vi "Get Edge Cost.vi"(8 "error in (no error)":errorcluster, 9 "end node":string, 10 "start node":string, 11 "map reference in":refnum<data-value>) -> (0 "error out":errorcluster, 1 "found?":bool, 2 "cost":dbl, 3 "map reference out":refnum<data-value>)   [LabVIEW 2017, in "NI_Robotics_DirectedGraphWorldMap.lvclass"]
doc: "Returns the cost of traversing the edge, or area, of the directed graph map between <B>start node</B> and <B>end node</B>."
uses:
  <vilib>/robotics/Navigation/shared/WorldMap/DirectedGraphWorldMap/NI_Robotics_DirectedGraphWorldMap.lvclass
  <vilib>/robotics/Navigation/shared/MapNode/DirectedGraphMapNode/NI_Robotics_DirectedGraphMapNode.lvclass
  c:/Program Files (x86)/National Instruments/LabVIEW 2017/vi.lib/robotics/Navigation/shared/MapNode/AbstractMapNode/NI_Robotics_AbstractMapNode.lvclass
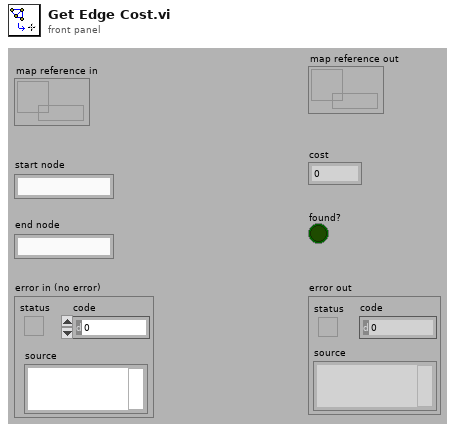
[diagram p1: front panel]
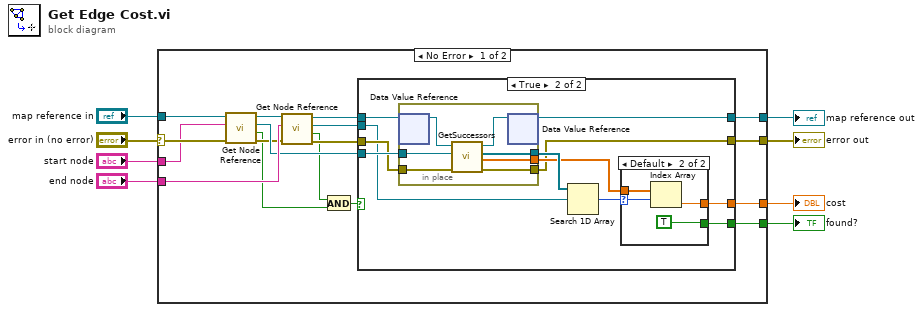
[diagram p0: block diagram]
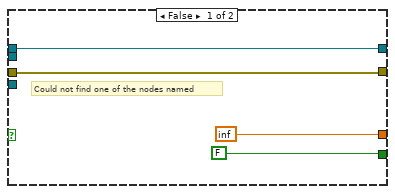
[diagram p2: hidden frame]
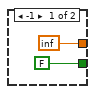
[diagram p3: hidden frame]
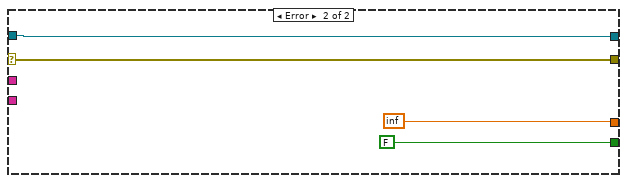
[diagram p4: hidden frame]
diagram:
  n1 = case shown="No Error" "error in (no error)" {
    selector: "error in (no error)" -> [w24 w56]
    tunnel: "map reference in" -> [w25 w57]
    tunnel: "start node" -> [w23 _]
    tunnel: "end node" -> [w21 _]
    tunnel: [w12 w57] -> w2
    tunnel: [w11 inf] -> w4
    tunnel: [w10 w56] -> w5
    tunnel: [w9 FALSE ("found?")] -> w1
    frame No Error {
      n2 = call <vilib>:"Get Node Reference.vi"("error in (no error)"=w24, "name"=w23, "map reference in"=w25) -> ("error out"=w17:errorcluster, "found?"=w13:bool, "node reference"=w19:refnum<data-value>, "map reference out"=w22:refnum<data-value>)  [unwired: 5 in]
      n3 = call <vilib>:"Get Node Reference.vi"("error in (no error)"=w17, "name"=w21, "map reference in"=w22) -> ("error out"=w16:errorcluster, "found?"=w14:bool, "node reference"=w18:refnum<data-value>, "map reference out"=w20:refnum<data-value>)  [unwired: 5 in]
      n4 = And(x=w14, y=w13) -> (x .and. y?=w15:bool)
      n5 = case shown="True" w15 {
        tunnel: w20 -> [w29 w33]
        tunnel: w19 -> [_ w40]
        tunnel: w18 -> [_ w34]
        tunnel: w16 -> [w26 w39]
        tunnel: [w26 w30] -> w10
        tunnel: [w29 w32] -> w12
        tunnel: [inf w35] -> w11
        tunnel: [FALSE ("found?") w31] -> w9
        frame False {
          # "Could not find one of the nodes named"
        }
        frame True {
          n6 = in-place {
            in-place-border: w40 -> [w47]
            in-place-border: w39 -> [w46]
            in-place-border: [w45] -> w30
            in-place-border: [w44] -> w37
            in-place-border: [w43] -> w36
            n7 = in-place-dvr #1(w33) -> (w42:refnum<class "NI_Robotics_DirectedGraphWorldMap.lvclass">)  [unwired: 1 out]
            n8 = call-dynamic "GetSuccessors.vi"("error in (no error)"=w46, "AbstractMapNode Ref"=w47, "WorldMap in"=w42) -> ("error out"=w45:errorcluster, "EdgeCost"=w43:dbl[], "Successors"=w44:refnum<data-value>[], "WorldMap out"=w41:refnum<class "NI_Robotics_DirectedGraphWorldMap.lvclass">)  [unwired: 5 in]
            n9 = in-place-dvr #1(w41) -> (w32:refnum<data-value>)  [unwired: 1 out]
          }
          n10 = Search 1D Array(1D array=w37, element=w34) -> (index of element=w38:i32)  [unwired: 1 in]
          n11 = case shown="Default" w38 {
            selector: w38 -> [_ w53]
            tunnel: w36 -> [_ w52]
            tunnel: [inf w51] -> w35
            tunnel: [FALSE ("found?") TRUE ("found?")] -> w31
            frame -1 {
            }
            frame Default {
              n12 = Index Array(array=w52, index=w53) -> (element=w51:dbl)
            }
          }
        }
      }
    }
    frame Error {
    }
  }
  "error out" <- w5
  "cost" <- w4
  "map reference out" <- w2
  "found?" <- w1
